vi "Read Power Setpoint (Array).vi"(8 "error in":errorcluster, 11 "Power Control in":refnum<class "Power Control.lvclass">) -> (0 "error out":errorcluster, 1 "Changed or First Call?":bool, 2 "Power Setpoint":dbl[](array[numeric]), 3 "Power Control out":refnum<class "Power Control.lvclass">)   [LabVIEW 2023, in "Power Control.lvclass"]
uses:
  Power Control.lvclass
  Power Control.lvclass/Power Control.ctl
  af94bebd-7708-4158-8814-30f53347f523.vi
  <vilib>/ADAS Replay HIL/Channels/Tag Wrapper/Polymorphic/Read Channel (Double).vi/b2f764de-0c1e-4784-a155-687fc995a684.vi
  <vilib>/ADAS Replay HIL/Channels/Tag Wrapper/Polymorphic/Read Channel (Double).vi/b2f764de-0c1e-4784-a155-687fc995a684.vi/c28b0ead-42ad-4072-80a2-aca7f2bd7ce3.vi
  <vilib>/ADAS Replay HIL/Channels/Tag Wrapper/Polymorphic/Read Channel (Double).vi/b2f764de-0c1e-4784-a155-687fc995a684.vi/219d0231-d98b-4193-b5cc-84f90e3c9091.vi
  <vilib>/ADAS Replay HIL/Channels/Tag Wrapper/Polymorphic/Read Channel (Double).vi
  <vilib>/ADAS Replay HIL/Channels/Tag Wrapper/Tag Wrapper.lvlib
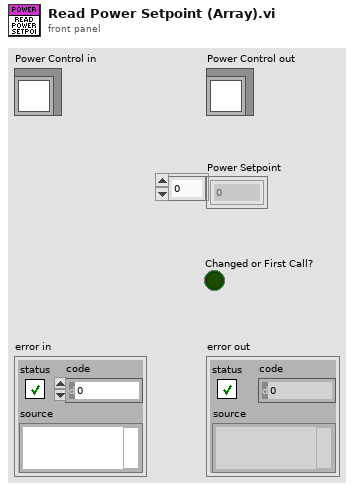
[diagram p1: front panel]
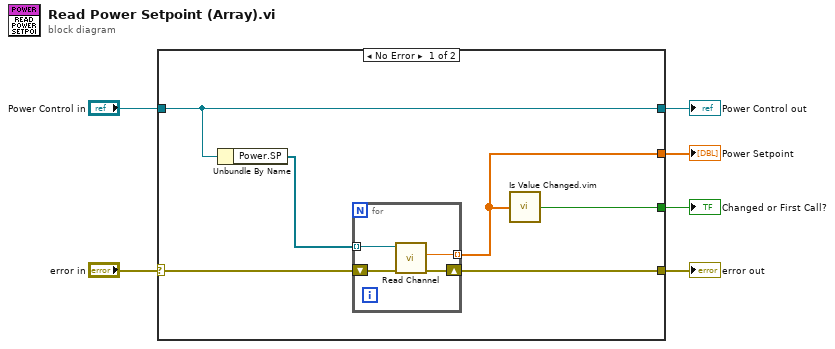
[diagram p0: block diagram]
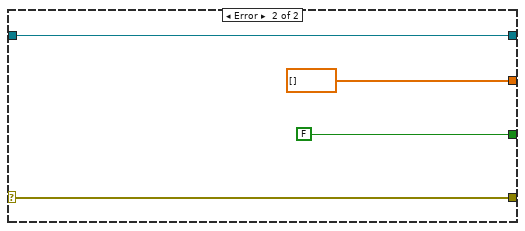
[diagram p2: hidden frame]
diagram:
  n1 = case shown="No Error" "error in" {
    selector: "error in" -> [w12 w20]
    tunnel: [w10 w20] -> w5
    tunnel: [w11 w19] -> w3
    tunnel: "Power Control in" -> [w11 w19]
    tunnel: [w8 dbl[] []] -> w2
    tunnel: [w7 FALSE ("changed or first call?")] -> w1
    frame No Error {
      n2 = Unbundle By Name(w11) -> ("Power.SP"=w9:refnum<k21>[])
      n3 = for {
        tunnel: w9 -> [w14] mode=indexing
        tunnel: [w13] -> w8 mode=indexing
        shift-right: [w15] -> w10
        shift-left: w12 -> [w16]
        n4 = call-poly <vilib>:"Read Channel.vi"("error in"=w16, "ADAS HIL Channel in"=w14) -> ("error out"=w15:errorcluster, "Value out"=w13:dbl)  [unwired: 6 in, 2 out]
      }
      n5 = call "Is Value Changed.vim"("value"=w8) -> ("changed or first call?"=w7:bool)
    }
    frame Error {
    }
  }
  "error out" <- w5
  "Power Control out" <- w3
  "Power Setpoint" <- w2
  "Changed or First Call?" <- w1
